vi "GUI_Bella_IP2_LiquidCrystal.vi"() -> ()   [LabVIEW 2020]
uses:
  Shared/GUI_Template/GUI_master/tcp_new_data_event.ctl
  Shared/GUI_Template/GUI_master/tcp new data cluster.ctl
  <vilib>/vision/Image Controls.llb/IMAQ Image.ctl
panel:
  in  "save::2":bool caption="Trigger"
  in  "delay.Channel_B::3":dbl=0.005 caption="delay B" min=-0.1 max=0.1 format="%.3p"
  in  "GUIdevice 3":string="P2-DG535" caption="GUIdevice 4"
  in  "Min Threshold":dbl
  in  "Manual Shutter Controls":bool
  in  "Shot Mode":bool
  in  "fwhmy::1":dbl caption="Max Counts" min=0.0 max=999999.0
  in  "fwhmx::1":dbl caption="Max Counts" min=0.0 max=999999.0
  out "Film in place?":bool
  in  "fwhmx::1":dbl caption="Max Counts" min=0.0 max=999999.0
  in  "Min Threshold":dbl
  in  "trigger::1":bool caption="Trigger"
  in  "trigger::2":bool caption="Trigger"
  in  "exposure::2":dbl=0.005 caption="exposure" min=3.8e-05 max=10.0 format="%.3p"
  in  "Target.X::2":dbl=200.0 caption="X" min=0.0 max=2000.0
  in  "Target.Y::2":dbl=200.0 caption="Y" min=0.0 max=2000.0
  in  "TargetSize.X::2":dbl=50.0 caption="Size X" min=2.0 max=3000.0
  in  "Color 2":u32(colorbox)=16711680 caption="Color"
  in  "TargetSize.Y::2":dbl=50.0 caption="Size Y" min=2.0 max=3000.0
  in  "Thickness 2":u8=3
  out "SideViewNorth":T1(plugin-control)
  in  "exposure::1":dbl=0.001 caption="exposure" min=3.8e-06 max=1.0 format="%.3p"
  out "Windmill_FF":T1(plugin-control)
  in  "Target.X::1":dbl=838.0 caption="X" min=0.0 max=2000.0
  in  "Target.Y::1":dbl=620.0 caption="Y" min=0.0 max=2000.0
  in  "TargetSize.X::1":dbl=50.0 caption="Size X" min=2.0 max=3000.0
  in  "Color 1":u32(colorbox)=16711680 caption="Color"
  in  "TargetSize.Y::1":dbl=50.0 caption="Size Y" min=2.0 max=3000.0
  in  "Thickness 1":u8=3
  in  "GUIdevice 2":string="P2_windmillTemp" caption="GUIdevice 4"
  out "image::2":T1(plugin-control) caption="M1 Cam"
  out "image::1":T1(plugin-control) caption="M1 Cam"
  in  "GUIdevice 1":string="P2-Windmill_FF" caption="GUIdevice 4"
  out "tcp data event":T2
  in  "stop":bool
  out "error IO 2":errorcluster
  # "Plasma2 LC Windmill CNTRL"
  # "Open"
  # "Automatic"
  # "Manual"
  # "Closed"
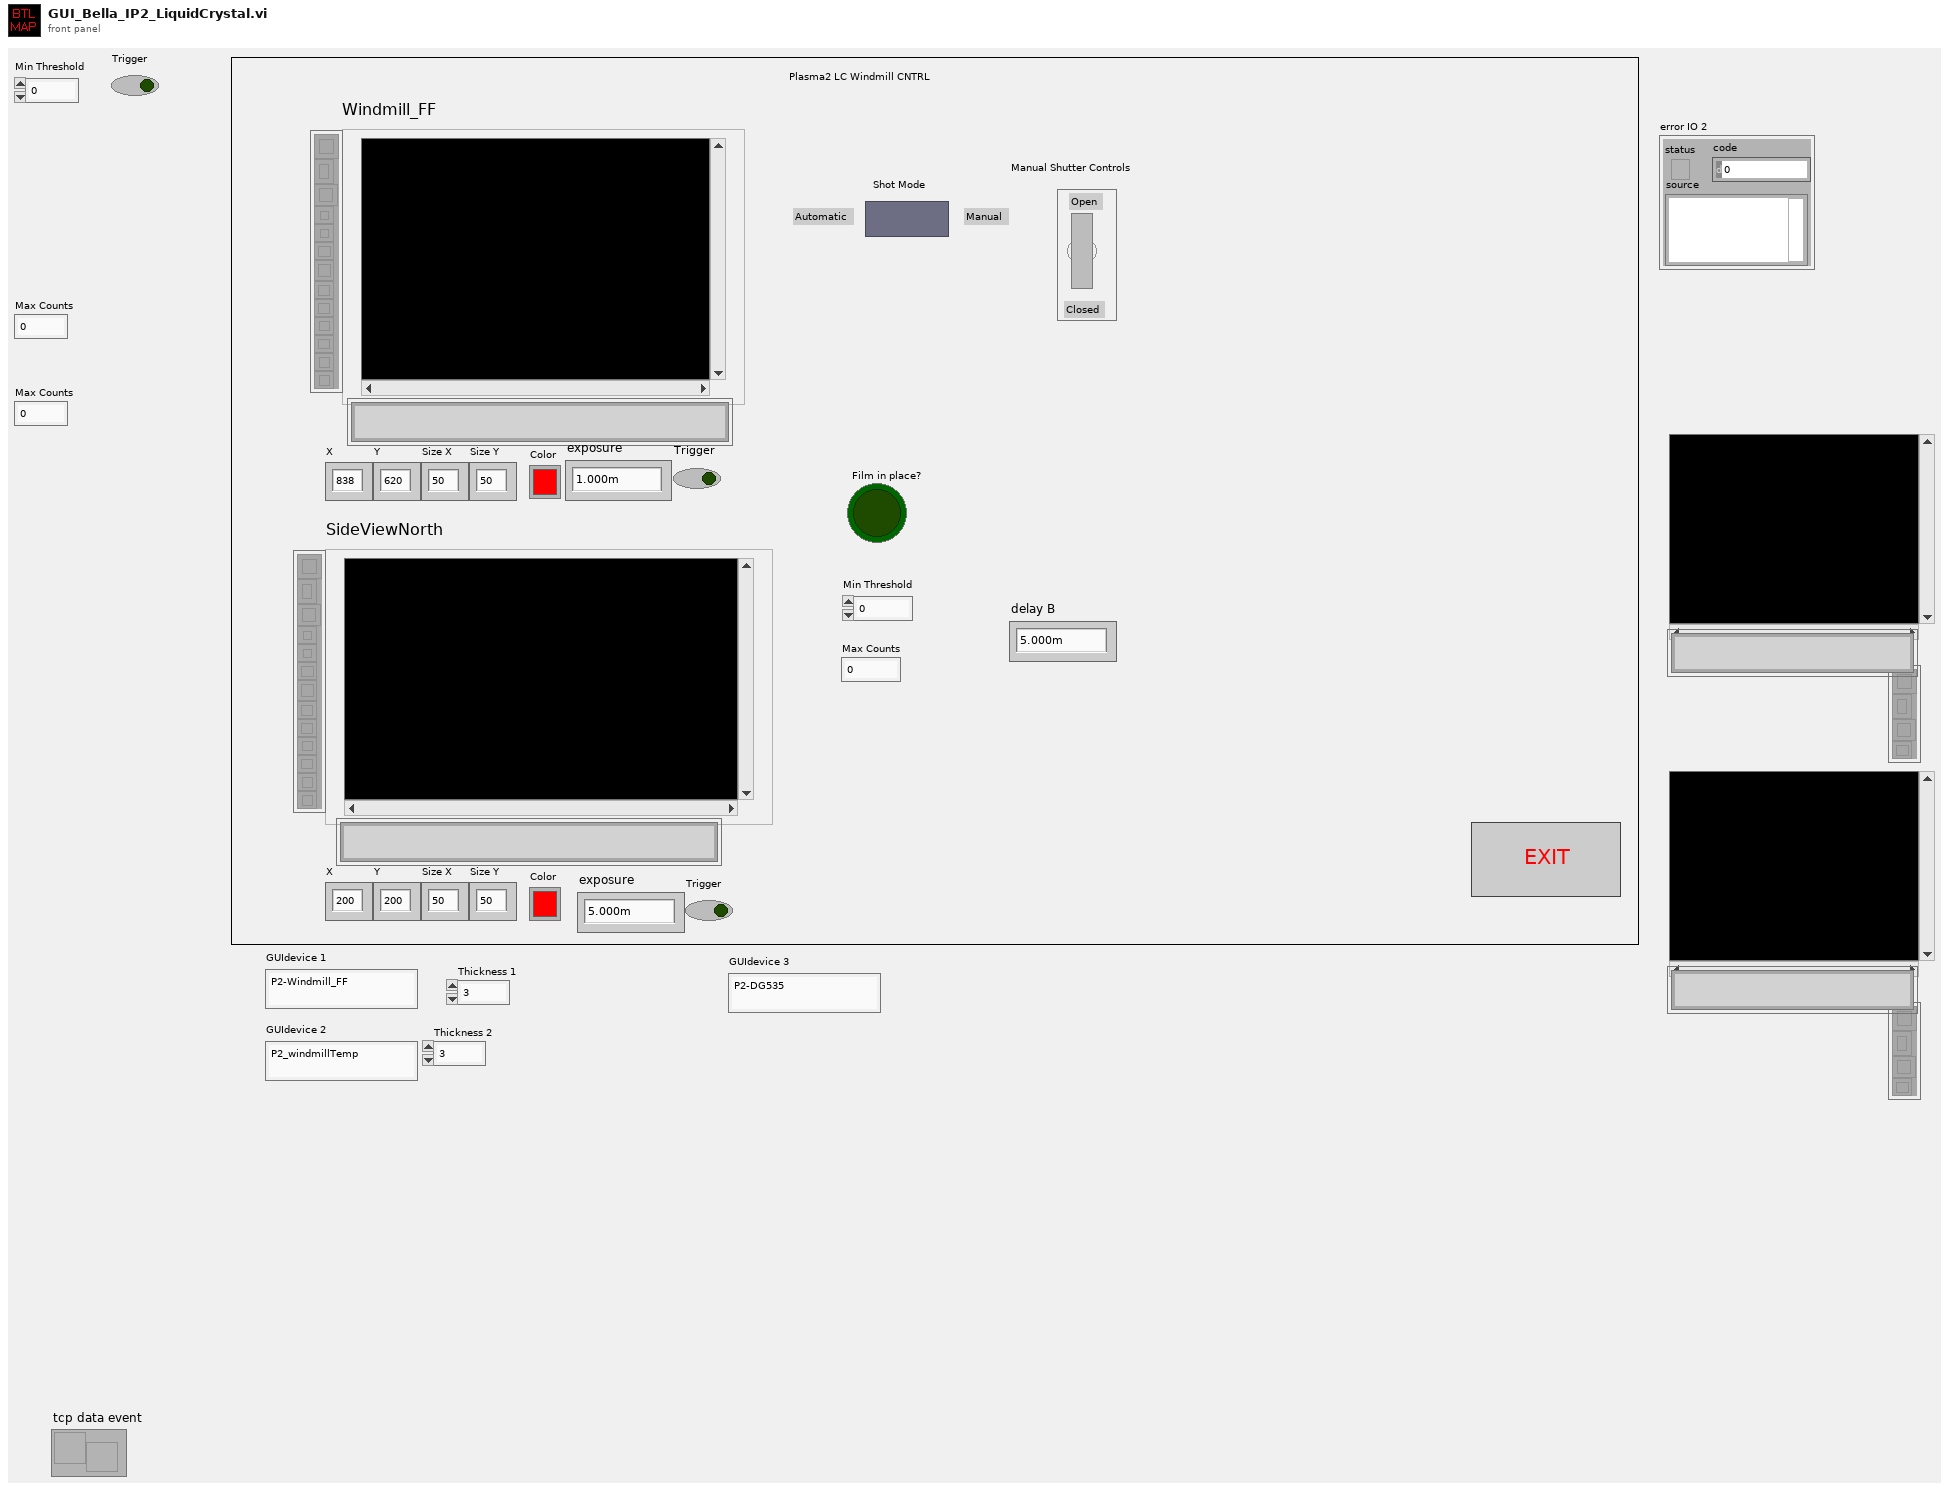
[diagram p1: front panel]
types:
  T1 = typedef "IMAQ Image.ctl" = refnum<image>
  T2 = typedef "tcp_new_data_event.ctl" = refnum<user-event>
  T3 = cluster{"Last update Cam1":u32, "Last update Cam2":u32, "Last update Cam3":u32, "Last update Cam4":u32, "Last update Cam5":u32, "Last update Cam6":u32, "Last update Cam7":u32, "Last update Cam8":u32}
  T4 = typedef "Image Type" = u32
  T5 = typedef "tcp new data cluster.ctl" = cluster{"EventEnum":enum16{"new data", "connection status update"}, "Device name":string}
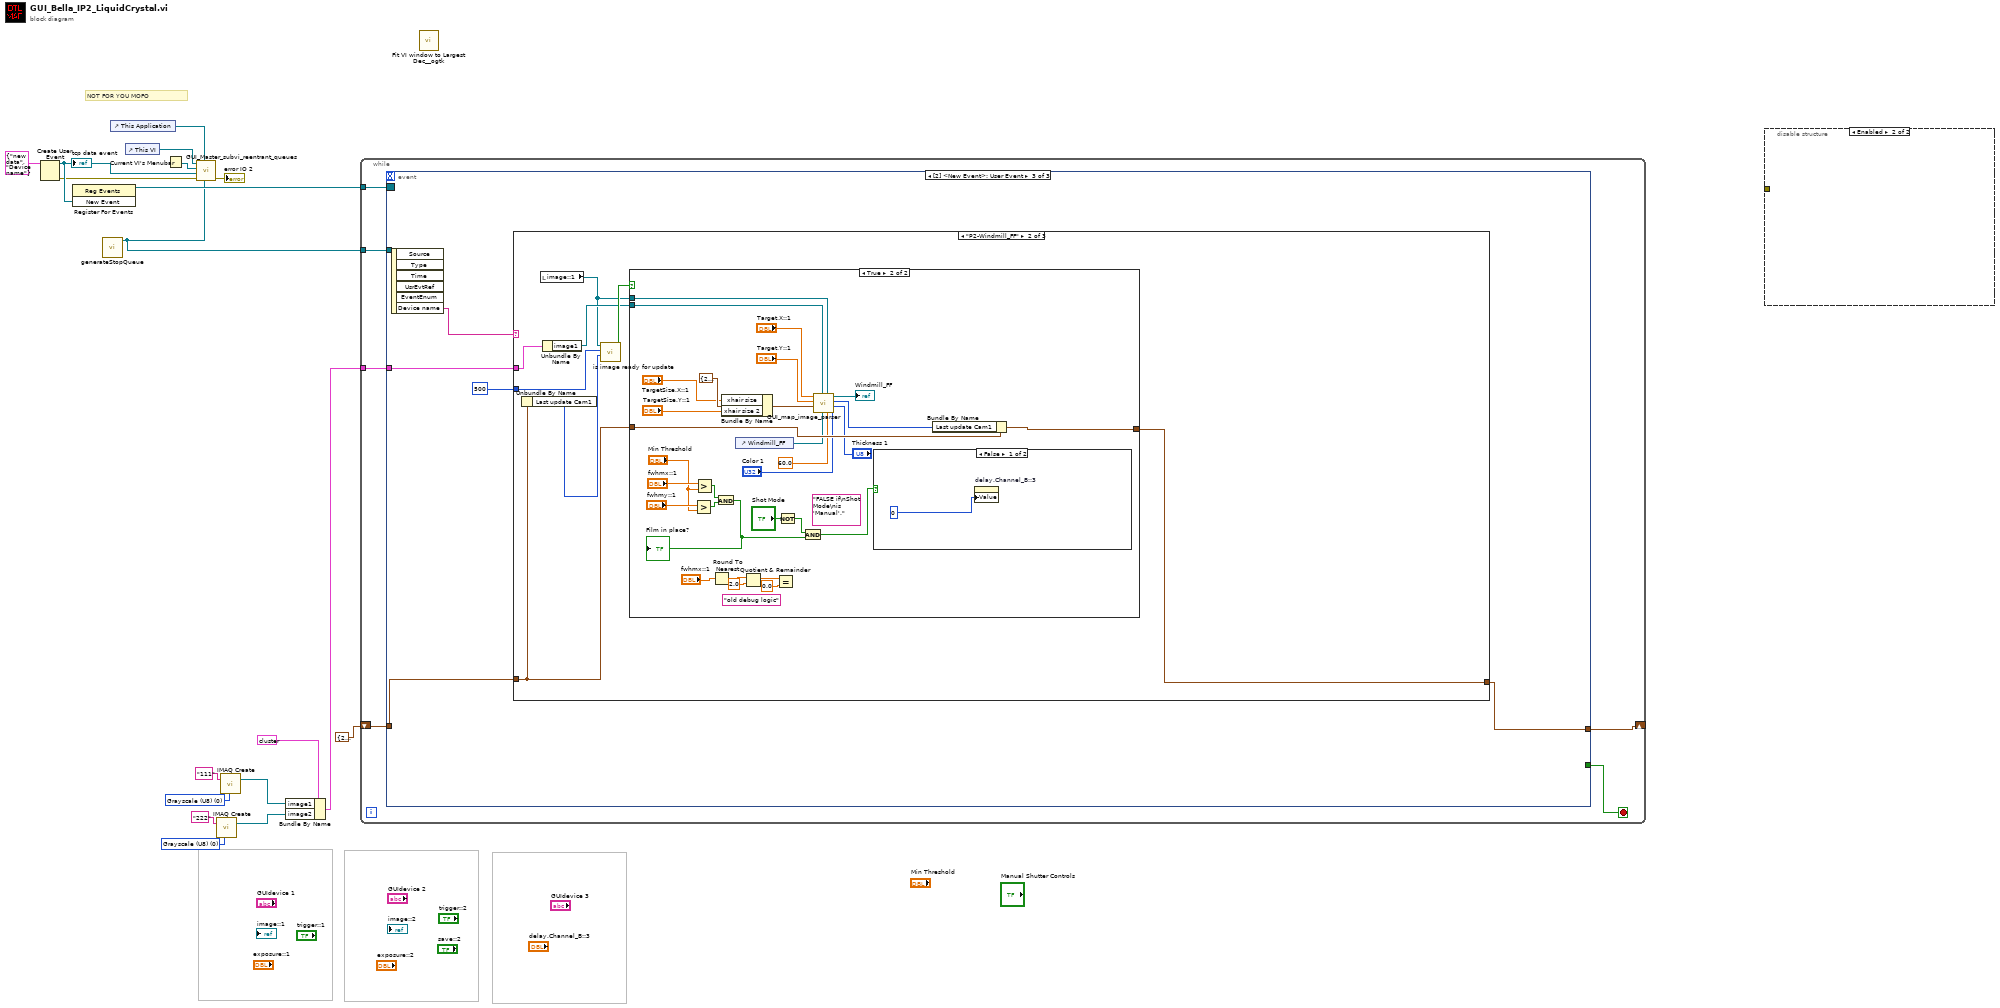
[diagram p0: block diagram]
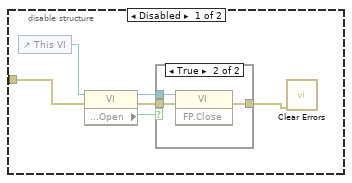
[diagram p2: hidden frame]
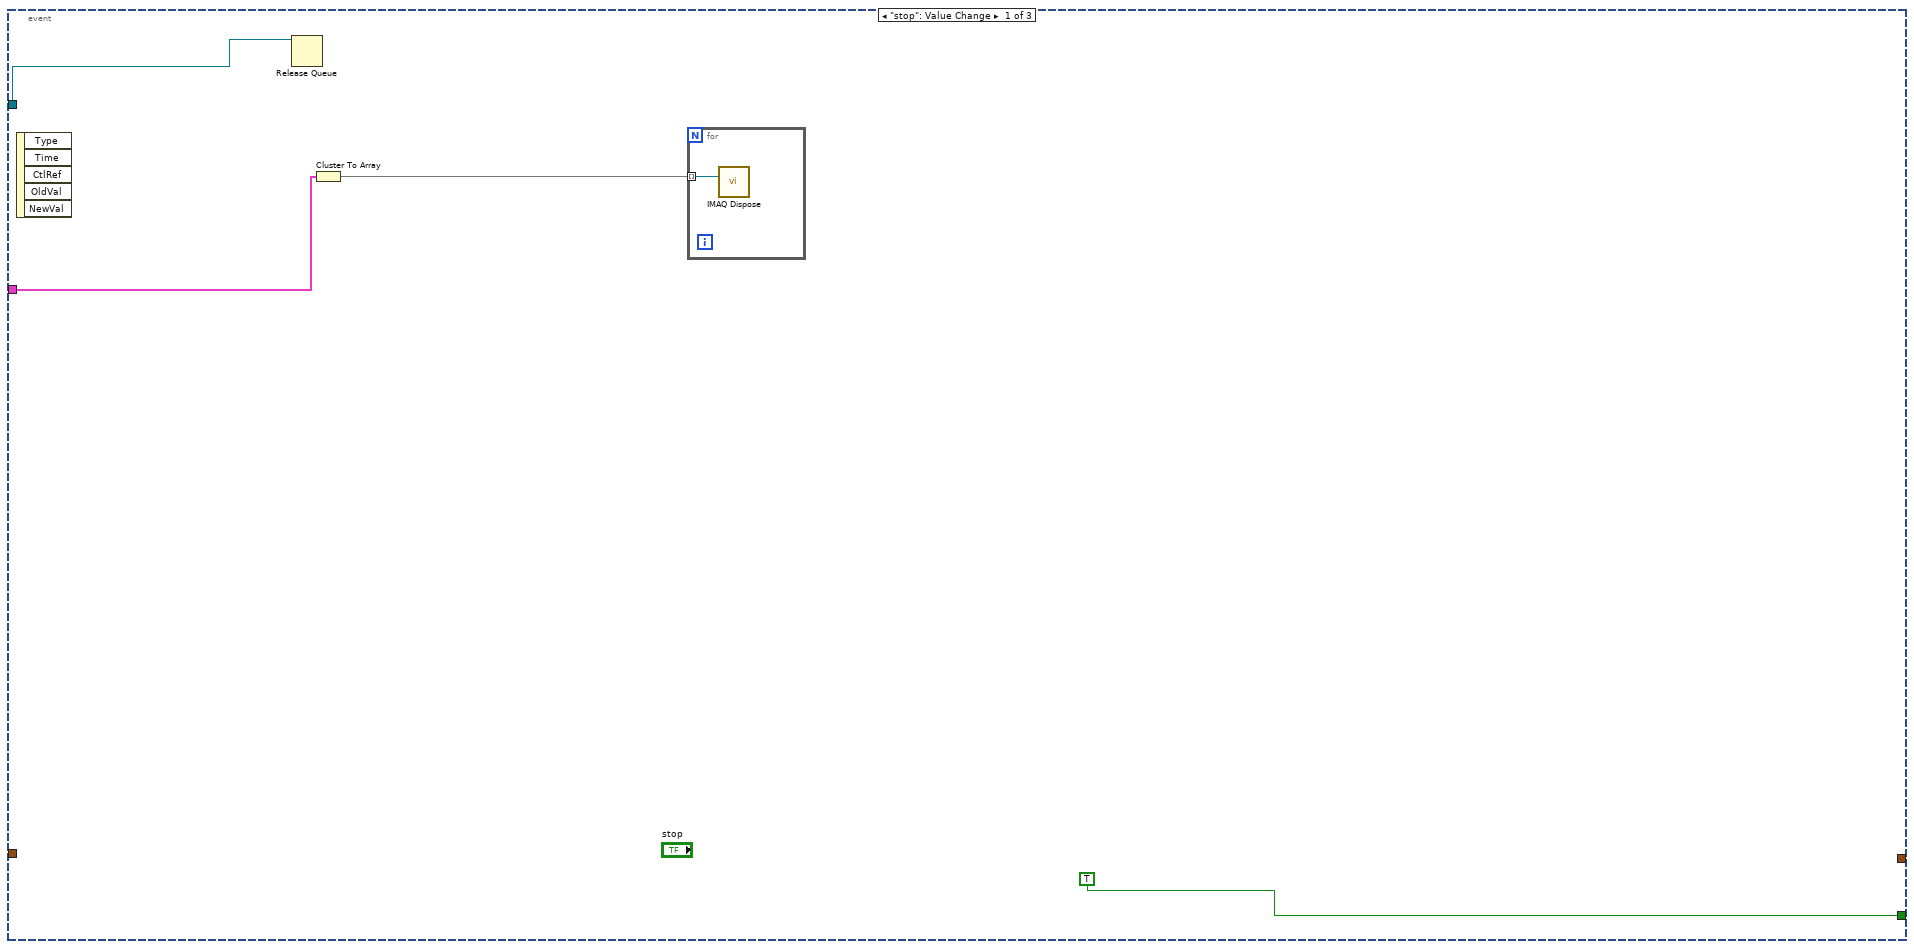
[diagram p4: hidden frame]
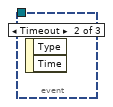
[diagram p5: hidden frame]
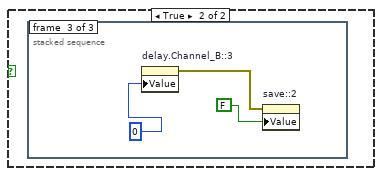
[diagram p8: hidden frame]
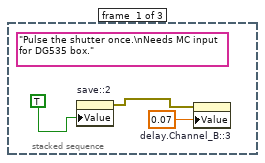
[diagram p9: hidden frame]
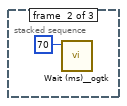
[diagram p10: hidden frame]
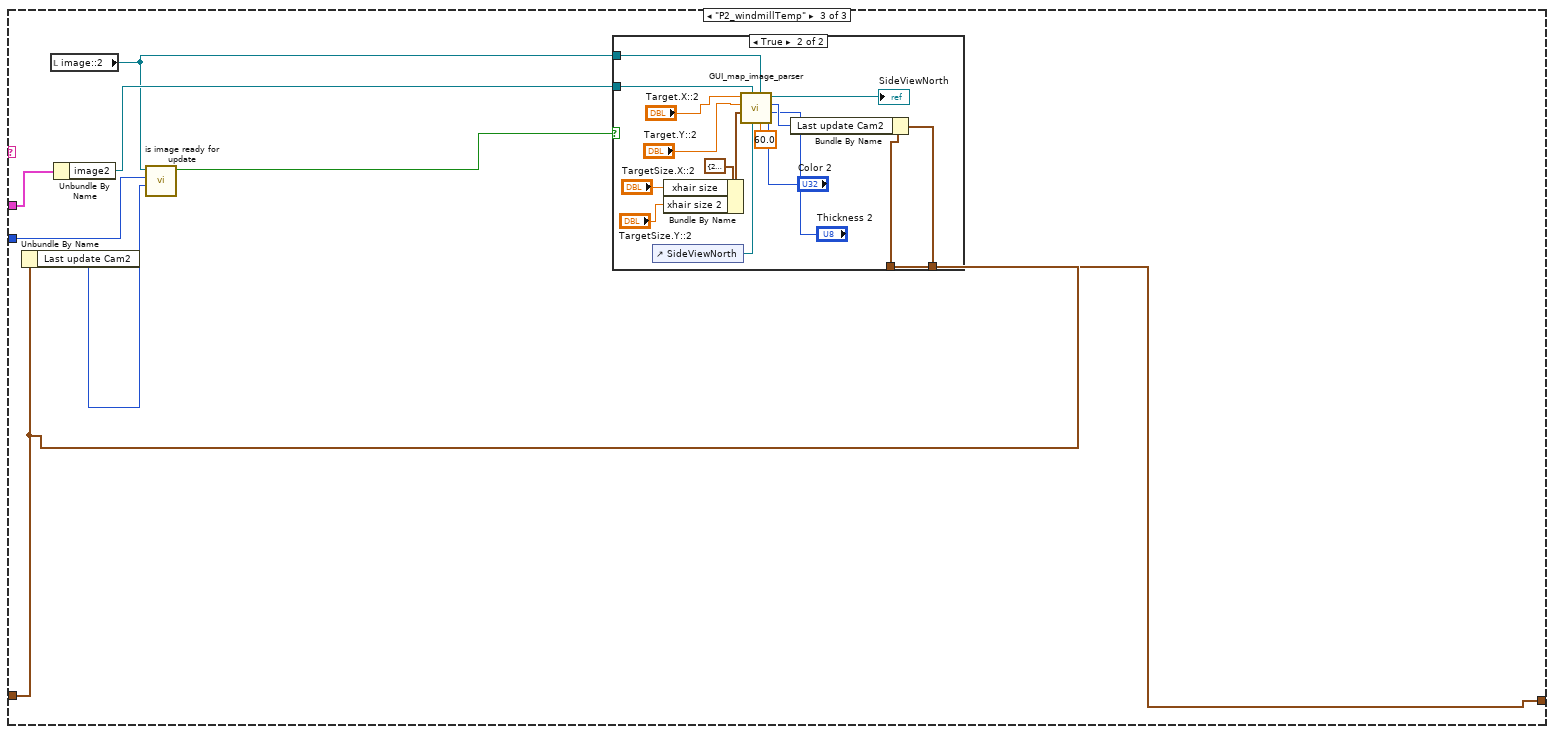
[diagram p11: hidden frame]
diagram:
  w8 = T4 0 items=["Grayscale (U8)", "Grayscale (I16)", "Grayscale (SGL)", "Complex (CSG)", "RGB (U32)", "HSL (U32)", "RGB (U64)", "Grayscale (U16)"] ("Image Type")
  w10 = T4 0 items=["Grayscale (U8)", "Grayscale (I16)", "Grayscale (SGL)", "Complex (CSG)", "RGB (U32)", "HSL (U32)", "RGB (U64)", "Grayscale (U16)"] ("Image Type")
  # "NOT FOR YOU MOFO"
  n1 = Create User Event(user event datatype=T5 {"EventEnum"=enum."new data", "Device name"="Device name"} ("New Event")) -> (user event=w17:refnum<user-event>, error out=w16:errorcluster)  [unwired: 1 in]
  "tcp data event" <- w17
  n2 = register-events(w17) -> (reference out=w11:refnum<event-registration>)  [unwired: 2 in, 1 out]
  n3 = call "generateStopQueue.vi"() -> ("STOP Queue out"=w1:refnum<queue>)  [unwired: 10 in, 1 out]
  n4 = control-ref of="This Application"() -> (w18:refnum<vi>)
  n5 = control-ref of="This VI"() -> (w13:refnum<vi>)
  n6 = Current VI's Menubar() -> (w14:refnum<k9>)
  n7 = call "GUI_Master_subvi_reentrant_queues.vi"("STOP Queue in"=w1, "This Application"=w18, "error in (no error)"=w16, "tcp data event"=w17, "Caller menu reference"=w14, "Caller VI ref"=w13) -> ("error out"=→"error IO 2":errorcluster)  [unwired: 5 in]
  n8 = call "IMAQ Create"("Image Name"="222", "Image Type"=w10) -> ("New Image"=w5:T1)  [unwired: 3 in, 1 out]
  n9 = call "IMAQ Create"("Image Name"="111", "Image Type"=w8) -> ("New Image"=w6:T1)  [unwired: 3 in, 1 out]
  n10 = Bundle By Name(cluster=cluster{"image1":T1, "image2":T1} {"image1"="image1", "image2"="image2"} ("input cluster"), "image1"=w6, "image2"=w5) -> (w3:cluster{"image1":T1, "image2":T1})
  n11 = while {
    tunnel: w11 -> [w23]
    tunnel: w3 -> [w22]
    shift-right: [w20] -> _
    shift-left: T3 {"Last update Cam1"=200, "Last update Cam2"=200, "Last update Cam3"=200, "Last update Cam4"=200, "Last update Cam5"=200, "Last update Cam6"=200, "Last update Cam7"=200, "Last update Cam8"=200} -> [w21]
    tunnel: w1 -> [w19]
    stop <- w24 stop-if-true
    n12 = event shown="[2] <New Event>: User Event" {
      selector: w23 -> [_ _ _]
      dyn-events: _ -> [_ _ _]
      timeout: _ -> [_ _ _]
      tunnel: [TRUE ("stop") _ _] -> w24
      tunnel: w22 -> [w25 _ w33]
      tunnel: w21 -> [_ _ w32]
      tunnel: [_ _ w31] -> w20
      tunnel: w19 -> [w27 _ _]
      event "stop": Value Change {
        n13 = event-data() -> ()  [unwired: 1 in, 5 out]
        n14 = Release Queue(queue=w27) -> ()  [unwired: 2 in, 3 out]
        n15 = Cluster To Array(cluster=w25) -> (array=w26:T1[])
        n16 = for {
          tunnel: w26 -> [w29] mode=indexing
          n17 = call "IMAQ Dispose"("Image"=w29) -> ()  [unwired: 5 in, 1 out]
        }
      }
      event Timeout {
        n18 = event-data() -> ()  [unwired: 1 in, 2 out]
      }
      event User Event {
        n19 = event-data() -> ("Device name"=w34:string)  [unwired: 1 in, 5 out]
        n20 = case shown="\"P2-Windmill_FF\"" w34 {
          tunnel: w33 -> [_ w39 w86]
          tunnel: w32 -> [w35 w41 w88]
          tunnel: [w35 w40 w87] -> w31
          tunnel: u32 500 ("x-y") -> [_ w36 w83]
          frame "False", Default {
          }
          frame "P2-Windmill_FF" {
            n21 = Unbundle By Name(w41) -> ("Last update Cam1"=w42:u32)
            n22 = local read "image::1"() -> (w37:T1)
            n23 = Unbundle By Name(w39) -> ("image1"=w38:T1)
            n24 = call "is image ready for update.vi"("Last update"=w42, "min time between updates"=w36, "image ref in"=w37) -> ("update image"=w43:bool)  [unwired: 8 in]
            n25 = case shown="True" w43 {
              tunnel: w41 -> [w44 w74]
              tunnel: [w44 w73] -> w40
              tunnel: w37 -> [_ w72]
              tunnel: w38 -> [_ w64]
              frame False {
              }
              frame True {
                (unwired) "old debug logic"
                (unwired) "FALSE if\nShot Mode\nis 'Manual'."
                n26 = Greater?(x="fwhmy::1", y="Min Threshold") -> (0:w52:bool)
                n27 = Greater?(x="fwhmx::1", y="Min Threshold") -> (0:w51:bool)
                n28 = Round To Nearest(number="fwhmx::1") -> (nearest integer value=w57:dbl)
                n29 = And(x=w51, y=w52) -> (x .and. y?=w47:bool)
                "Film in place?" <- w47
                n30 = Bundle By Name(cluster=cluster{"xhair size":dbl, "xhair size 2":dbl} {"xhair size"=20.0, "xhair size 2"=20.0} ("size"), "xhair size"="TargetSize.X::1", "xhair size 2"="TargetSize.Y::1") -> (w65:cluster{"xhair size":dbl, "xhair size 2":dbl})
                n31 = control-ref of="Windmill_FF"() -> (w59:refnum<vi>)
                n32 = Quotient & Remainder(x=w57, y=2.0) -> (x-y*floor(x/y)=w56:dbl)  [unwired: 1 out]
                n33 = Equal?(x=w56, y=0.0) -> ()  [unwired: 1 out]
                n34 = Not(x="Shot Mode") -> (.not. x?=w49:bool)
                n35 = And(x=w49, y=w47) -> (x .and. y?=w45:bool)
                n36 = call "GUI_map_image_parser.vi"("color"="Color 1", "Thickness"="Thickness 1", "zoom#"=60.0, "Image Src"=w72, "Ctl Refnum"=w59, "Image Dst"=w64, "size"=w65, "target y"="Target.Y::1", "target x"="Target.X::1") -> ("ms timer out"=w69:u32, "Img out"=→"Windmill_FF":T1)  [unwired: 1 in]
                n37 = case shown="False" w45 {
                  frame False {
                    n38 = property on="delay.Channel_B::3" class="DigNum (strict)"("Value"=0) -> ()  [unwired: 2 in, 2 out]
                  }
                  frame True {
                    n39 = stacked-sequence {
                      frame #0 {
                        (unwired) "Pulse the shutter once.\nNeeds MC input for DG535 box."
                        n40 = property on="save::2" class="Bool (strict)"("Value"=TRUE) -> (error out=w76:errorcluster)  [unwired: 2 in, 1 out]
                        n41 = property on="delay.Channel_B::3" class="DigNum (strict)"(error in=w76, "Value"=0.07) -> ()  [unwired: 1 in, 2 out]
                      }
                      frame #1 {
                        n42 = call <userlib>:"Wait (ms)__ogtk.vi"("milliseconds to wait"=u32 70) -> ()  [unwired: 9 in, 2 out]
                      }
                      frame #2 {
                        n43 = property on="delay.Channel_B::3" class="DigNum (strict)"("Value"=0) -> (error out=w80:errorcluster)  [unwired: 2 in, 1 out]
                        n44 = property on="save::2" class="Bool (strict)"(error in=w80, "Value"=FALSE) -> ()  [unwired: 1 in, 2 out]
                      }
                    }
                  }
                }
                n45 = Bundle By Name(cluster=w74, "Last update Cam1"=w69) -> (w73:T3)
              }
            }
          }
          frame "P2_windmillTemp" {
            n46 = Unbundle By Name(w88) -> ("Last update Cam2"=w89:u32)
            n47 = local read "image::2"() -> (w84:T1)
            n48 = Unbundle By Name(w86) -> ("image2"=w85:T1)
            n49 = call "is image ready for update.vi"("Last update"=w89, "min time between updates"=w83, "image ref in"=w84) -> ("update image"=w90:bool)  [unwired: 8 in]
            n50 = case shown="True" w90 {
              tunnel: w88 -> [w91 w107]
              tunnel: [w91 w106] -> w87
              tunnel: w84 -> [_ w105]
              tunnel: w85 -> [_ w97]
              frame False {
              }
              frame True {
                n51 = control-ref of="SideViewNorth"() -> (w92:refnum<vi>)
                n52 = Bundle By Name(cluster=cluster{"xhair size":dbl, "xhair size 2":dbl} {"xhair size"=20.0, "xhair size 2"=20.0} ("size"), "xhair size"="TargetSize.X::2", "xhair size 2"="TargetSize.Y::2") -> (w98:cluster{"xhair size":dbl, "xhair size 2":dbl})
                n53 = call "GUI_map_image_parser.vi"("color"="Color 2", "Thickness"="Thickness 2", "zoom#"=60.0, "Image Src"=w105, "Ctl Refnum"=w92, "Image Dst"=w97, "size"=w98, "target y"="Target.Y::2", "target x"="Target.X::2") -> ("ms timer out"=w102:u32, "Img out"=→"SideViewNorth":T1)  [unwired: 1 in]
                n54 = Bundle By Name(cluster=w107, "Last update Cam2"=w102) -> (w106:T3)
              }
            }
          }
        }
      }
    }
  }
  n55 = call <userlib>:"Fit VI window to Largest Dec__ogtk.vi"() -> ()  [unwired: 6 in, 2 out]
  n56 = disable-structure shown="Enabled" {
    disable-tunnel: _ -> [w109 _]
    frame Disabled {
      n57 = control-ref of="This VI"() -> (w110:refnum<vi>)
      n58 = property class="VI"(reference=w110, error in=w109) -> (reference out=w112:refnum<vi>, error out=w113:errorcluster, "Front Panel.Open"=w111:bool)
      n59 = case shown="True" w111 {
        tunnel: [w114 w117] -> w108
        tunnel: w113 -> [w114 w116]
        tunnel: w112 -> [_ w115]
        frame False {
        }
        frame True {
          n60 = invoke class="VI" method="FP.Close"(reference=w115, error in=w116) -> (error out=w117:errorcluster)  [unwired: 1 in, 2 out]
        }
      }
      n61 = call <vilib>:"Clear Errors.vi"("error in (no error)"=w108) -> ()  [unwired: 5 in, 2 out]
    }
    frame Enabled {
    }
  }
